vi "Save_scan_as_BMP(working).vi"() -> ()   [LabVIEW 2016]
uses:
  <vilib>/picture/picture.llb/imagedata.ctl
panel:
  in  "error in (no error)":errorcluster
  out "error out":errorcluster
  out "IsObj":bool
  out "BMP":picture
  in  "BMP MAIN FOLDER":path
  out "BMP Path":path
  in  "Application":refnum<k7>
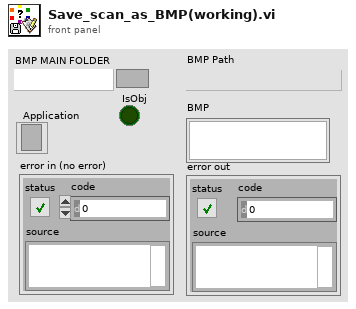
[diagram p1: front panel]
types:
  T1 = cluster{"left":i16, "top":i16, "right":i16, "bottom":i16}
  T2 = typedef "imagedata.ctl" = cluster{"image type":i32, "image depth":i32, "image":u8[], "mask":u8[], "colors":u32[], "Rectangle":cluster{"left":i16, "top":i16, "right":i16, "bottom":i16}}
  T3 = typedef "LVRectTypeDef.ctl" = cluster{"Left":i16, "Top":i16, "Right":i16, "Bottom":i16}
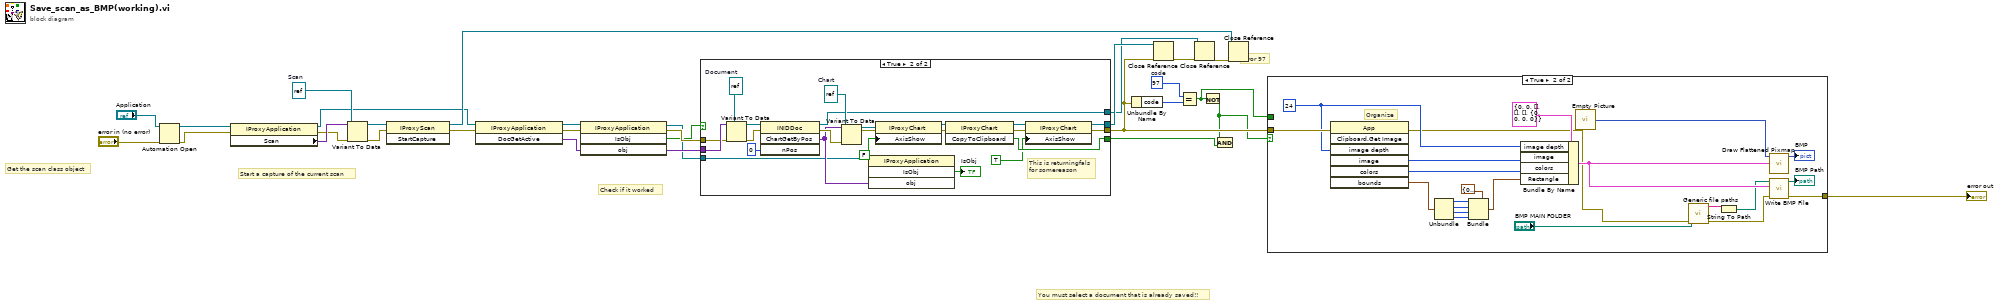
[diagram p0: block diagram]
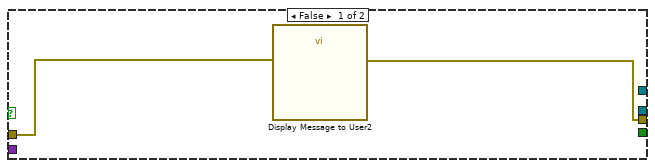
[diagram p2: hidden frame]
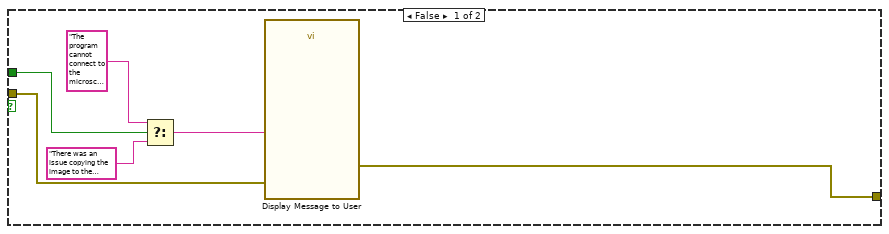
[diagram p3: hidden frame]
diagram:
  w8 = refnum<k7> refnum  # Scan
  w26 = 97  # code
  # "Check if it worked"
  # "Start a capture of the current scan"
  # "Get the scan class object"
  # "You must select a document that is already saved!!"
  # "Error 97"
  n1 = Automation Open(error in (no error)="error in (no error)", Automation Refnum="Application") -> (Automation Refnum=w11:refnum<k7>, error out=w10:errorcluster)  [unwired: 2 in]
  n2 = property class="IProxyApplication"(reference=w11, error in=w10) -> (reference out=w4:refnum<k7>, error out=w3:errorcluster, "Scan"=w14:variant)
  n3 = Variant To Data(error in=w3, type=w8, Variant=w14) -> (data=w13:refnum<k7>, error out=w12:errorcluster)
  n4 = invoke class="IProxyScan" method="StartCapture"(reference=w13, error in=w12) -> (reference out=w6:refnum<k7>, error out=w9:errorcluster)  [unwired: 1 in, 1 out]
  n5 = invoke class="IProxyApplication" method="DocGetActive"(reference=w4, error in=w9) -> (reference out=w30:refnum<k7>, error out=w27:errorcluster, "DocGetActive"=w20:variant)  [unwired: 1 in]
  n6 = invoke class="IProxyApplication" method="IsObj"(reference=w30, error in=w27, "obj"=w20) -> (reference out=w2:refnum<k7>, error out=w28:errorcluster, "IsObj"=w1:bool, "obj"=w29:variant)  [unwired: 1 in]
  n7 = case shown="True" w1 {
    tunnel: [_ w40] -> w24
    tunnel: w29 -> [_ w52]
    tunnel: w28 -> [w31 w51]
    tunnel: [w32 w41] -> w16
    tunnel: [_ w38] -> w19
    tunnel: [_ w37] -> w18
    tunnel: w2 -> [_ w34]
    frame False {
      n8 = call "Display Message to User2"("error in (no error)"=w31) -> ("error out"=w32:errorcluster)  [unwired: 9 in, 1 out]
    }
    frame True {
      w55 = refnum<k7> refnum  # Document
      w44 = refnum<k7> refnum  # Chart
      # "This is returningfals\nfor somereason"
      n9 = Variant To Data(error in=w51, type=w55, Variant=w52) -> (data=w54:refnum<k7>, error out=w53:errorcluster)
      n10 = invoke class="INIDDoc" method="ChartGetByPos"(reference=w54, error in=w53, "nPos"=0) -> (reference out=w37:refnum<k7>, error out=w50:errorcluster, "ChartGetByPos"=w36:variant)  [unwired: 1 in, 1 out]
      n11 = Variant To Data(error in=w50, type=w44, Variant=w36) -> (data=w49:refnum<k7>, error out=w46:errorcluster)
      n12 = invoke class="IProxyApplication" method="IsObj"(reference=w34, "obj"=w36) -> ("IsObj"=→"IsObj":bool)  [unwired: 2 in, 3 out]
      n13 = property class="IProxyChart"(reference=w49, error in=w46, "AxisShow"=FALSE) -> (reference out=w47:refnum<k7>, error out=w45:errorcluster)
      n14 = invoke class="IProxyChart" method="CopyToClipboard"(reference=w47, error in=w45) -> (reference out=w43:refnum<k7>, error out=w42:errorcluster, "CopyToClipboard"=w40:bool)  [unwired: 1 in]
      n15 = property class="IProxyChart"(reference=w43, error in=w42, "AxisShow"=TRUE) -> (reference out=w38:refnum<k7>, error out=w41:errorcluster)
    }
  }
  n16 = Unbundle By Name(w16) -> ("code"=w25:i32)
  n17 = Close Reference(reference=w19, error in (no error)=w16) -> (error out=w17:errorcluster)
  n18 = Equal?(x=w26, y=w25) -> (x = y?=w23:bool)
  n19 = Close Reference(reference=w18, error in (no error)=w17) -> (error out=w5:errorcluster)
  n20 = Not(x=w23) -> (.not. x?=w15:bool)
  n21 = And(x=w15, y=w24) -> ()  [unwired: 1 out]
  n22 = Close Reference(reference=w6, error in (no error)=w5) -> ()  [unwired: 1 out]
  n23 = case shown="True" w15 {
    tunnel: w16 -> [w61 w83]
    tunnel: w23 -> [w60 _]
    tunnel: [w56 w68] -> w22
    frame False {
      n24 = Select(t="The program cannot connect to the microscope API, please make sure to view the Access Codes before using the program.  If the program still does not work, then try exiting the control software, and then using  task manager to close out of the program fully.", s=w60, f="There was an issue copying the image to the clipboard, please export image manually. ") -> (s? t:f=w57:string)
      n25 = call "Display Message to User"("error in (no error)"=w61, "Message"=w57) -> ("error out"=w56:errorcluster)  [unwired: 8 in, 1 out]
    }
    frame True {
      w70 = 24 ("Image Depth")
      # "Organize"
      n26 = invoke class="App" method="Clipboard.Get Image"(error in=w83, "image depth"=w70) -> (error out=w64:errorcluster, "image"=w82:u8[], "colors"=w81:u32[], "bounds"=w73:T3)  [unwired: 5 in, 3 out]
      n27 = Unbundle(w73) -> ("Left"=w77:i16, "Top"=w76:i16, "Right"=w75:i16, "Bottom"=w74:i16)
      n28 = Bundle(cluster=T1 {"left"=0, "top"=0, "right"=0, "bottom"=0} ("Rectangle"), "left"=w77, "top"=w76, "right"=w75, "bottom"=w74) -> (w72:T1)
      n29 = Bundle By Name(cluster=T2 {"image type"=0, "image depth"=0, "image"=[], "mask"=[], "colors"=[], "Rectangle"={"left"=0, "top"=0, "right"=0, "bottom"=0}} ("image data"), "image depth"=w70, "image"=w82, "colors"=w81, "Rectangle"=w72) -> (w71:T2)
      n30 = call "Empty Picture"() -> ("empty picture"=w80:picture)
      n31 = call "Generic file paths.vi"("error in (no error)"=w64, "Parent Folder"="BMP MAIN FOLDER") -> ("error out"=w65:errorcluster, "BMP Path"=w63:string)  [unwired: 6 in, 2 out]
      n32 = String To Path(string=w63) -> (path=w62:path)
      n33 = call <vilib>:"Draw Flattened Pixmap.vi"("image data"=w71, "picture"=w80) -> ("new picture"=→"BMP":picture)  [unwired: 7 in]
      n34 = call <vilib>:"Write BMP File.vi"("error in (no error)"=w65, "image data"=w71, "path to BMP file"=w62) -> ("error out"=w68:errorcluster, "path"=→"BMP Path":path)  [unwired: 7 in]
    }
  }
  "error out" <- w22
